vi "PicoScope4000aSettings.vi"(0 "handle in":i16=16384, 3 "Trigger Settings":T3={"Trigger Enabled"=FALSE, "Trigger Source"=enum."Channel A", "Trigger Threshold (Volts/Probe units)"=0.0, "Trigger Direction"=2, "Trigger Delay (samples)"=0, "Auto Trigger Time (ms)"=1000} {"Trigger Direction" items=["Above", "Below", "Rising", "Falling", "Rising or Falling"]}, 4 "Max ADC value":i16=32767, 5 "error in":errorcluster, 6 "Channel A Settings":T2={"Enabled"=FALSE, "Coupling"=1, "Range"=6, "Analogue Offset"=0.0, "Bandwidth Limit"=0} {"Bandwidth Limit" items=["Full", "20kHz", "100kHz", "1MHz"]; "Range" items=["10 mV", "20 mV", "50 mV", "100 mV", "200 mV", "500 mV", "1 V", "2 V", "5 V", "10 V", "20 V", "50 V ", "100 V"]; "Coupling" items=["AC", "DC"]}, 7 "Channel E Settings":T2={"Enabled"=FALSE, "Coupling"=1, "Range"=6, "Analogue Offset"=0.0, "Bandwidth Limit"=0} {"Bandwidth Limit" items=["Full", "20kHz", "100kHz", "1MHz"]; "Range" items=["10 mV", "20 mV", "50 mV", "100 mV", "200 mV", "500 mV", "1 V", "2 V", "5 V", "10 V", "20 V", "50 V ", "100 V"]; "Coupling" items=["AC", "DC"]}, 8 "Channel B Settings":T2={"Enabled"=FALSE, "Coupling"=1, "Range"=6, "Analogue Offset"=0.0, "Bandwidth Limit"=0} {"Bandwidth Limit" items=["Full", "20kHz", "100kHz", "1MHz"]; "Range" items=["10 mV", "20 mV", "50 mV", "100 mV", "200 mV", "500 mV", "1 V", "2 V", "5 V", "10 V", "20 V", "50 V ", "100 V"]; "Coupling" items=["AC", "DC"]}, 9 "Channel F Settings":T2={"Enabled"=FALSE, "Coupling"=1, "Range"=6, "Analogue Offset"=0.0, "Bandwidth Limit"=0} {"Bandwidth Limit" items=["Full", "20kHz", "100kHz", "1MHz"]; "Range" items=["10 mV", "20 mV", "50 mV", "100 mV", "200 mV", "500 mV", "1 V", "2 V", "5 V", "10 V", "20 V", "50 V ", "100 V"]; "Coupling" items=["AC", "DC"]}, 10 "Channel C Settings":T2={"Enabled"=FALSE, "Coupling"=1, "Range"=6, "Analogue Offset"=0.0, "Bandwidth Limit"=0} {"Bandwidth Limit" items=["Full", "20kHz", "100kHz", "1MHz"]; "Range" items=["10 mV", "20 mV", "50 mV", "100 mV", "200 mV", "500 mV", "1 V", "2 V", "5 V", "10 V", "20 V", "50 V ", "100 V"]; "Coupling" items=["AC", "DC"]}, 11 "Channel G Settings":T2={"Enabled"=FALSE, "Coupling"=1, "Range"=6, "Analogue Offset"=0.0, "Bandwidth Limit"=0} {"Bandwidth Limit" items=["Full", "20kHz", "100kHz", "1MHz"]; "Range" items=["10 mV", "20 mV", "50 mV", "100 mV", "200 mV", "500 mV", "1 V", "2 V", "5 V", "10 V", "20 V", "50 V ", "100 V"]; "Coupling" items=["AC", "DC"]}, 12 "Channel D Settings":T2={"Enabled"=FALSE, "Coupling"=1, "Range"=6, "Analogue Offset"=0.0, "Bandwidth Limit"=0} {"Bandwidth Limit" items=["Full", "20kHz", "100kHz", "1MHz"]; "Range" items=["10 mV", "20 mV", "50 mV", "100 mV", "200 mV", "500 mV", "1 V", "2 V", "5 V", "10 V", "20 V", "50 V ", "100 V"]; "Coupling" items=["AC", "DC"]}, 13 "Channel H Settings":T2={"Enabled"=FALSE, "Coupling"=1, "Range"=6, "Analogue Offset"=0.0, "Bandwidth Limit"=0} {"Bandwidth Limit" items=["Full", "20kHz", "100kHz", "1MHz"]; "Range" items=["10 mV", "20 mV", "50 mV", "100 mV", "200 mV", "500 mV", "1 V", "2 V", "5 V", "10 V", "20 V", "50 V ", "100 V"]; "Coupling" items=["AC", "DC"]}, 18 "Unit Info":T1={"Driver Version"="2.1.82.3072", "USB Version"="2.0", "Hardware"="1", "Variant"="4444", "Batch and Serial"="ET311/0003", "Cal Date"="24Jan17", "Kernel Version"="1.0", "Digital HW Version"="1", "Analogue HW Version"="1", "Firmware 1"="1.7.5.0", "Firmware 2"="1.1.6.0", "Num. channels"=4}) -> (14 "handle out":i16=16384, 16 "Enabled array":i16[](array[numeric])=[1, 0, 0, 0, 0, 0, 0, 0], 19 "error out":errorcluster)   [LabVIEW 2010]
doc: "This VI is used to set up the oscilloscope. The inputs are clusters for setting channel and simple trigger settings. Advanced triggers can be set up using PicoScope3000aAdvancedTriggerSettings.vi"
uses:
  Program Files/Pico Technology/SDK/lib/ps4000a.dll
  PicoScope4000aAnalogChannelSettings.ctl
panel:
  # "Note Bandwith Limit not avaiable on all models"
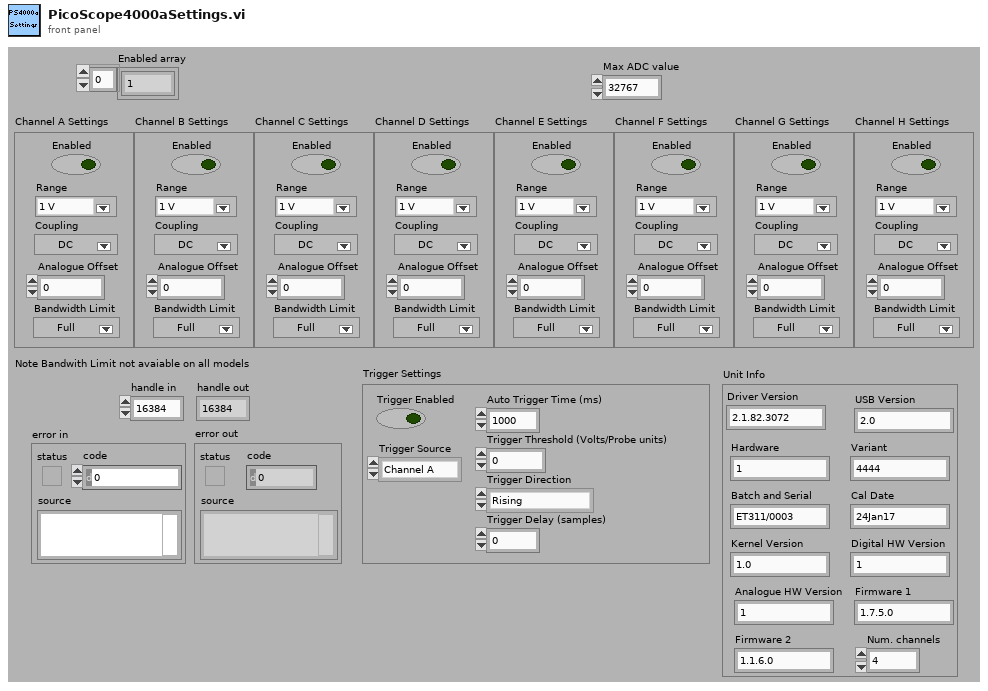
[diagram p1: front panel]
types:
  T1 = cluster{"Driver Version":string, "USB Version":string, "Hardware":string, "Variant":string, "Batch and Serial":string, "Cal Date":string, "Kernel Version":string, "Digital HW Version":string, "Analogue HW Version":string, "Firmware 1":string, "Firmware 2":string, "Num. channels":i16}
  T2 = typedef "PicoScope4000aAnalogChannelSettings.ctl" = cluster{"Enabled":bool, "Coupling":i16, "Range":u32, "Analogue Offset":sgl, "Bandwidth Limit":u32}
  T3 = cluster{"Trigger Enabled":bool, "Trigger Source":enum16{"Channel A", "Channel B", "Channel C", "Channel D", "Channel E", "Channel F", "Channel G", "Channel H"}, "Trigger Threshold (Volts/Probe units)":dbl, "Trigger Direction":u16, "Trigger Delay (samples)":u32, "Auto Trigger Time (ms)":i16}
  T4 = enum16{"Channel A", "Channel B", "Channel C", "Channel D", "Channel E", "Channel F", "Channel G", "Channel H"}
  T5 = cluster{"status":bool, "code":u32, "source":string}
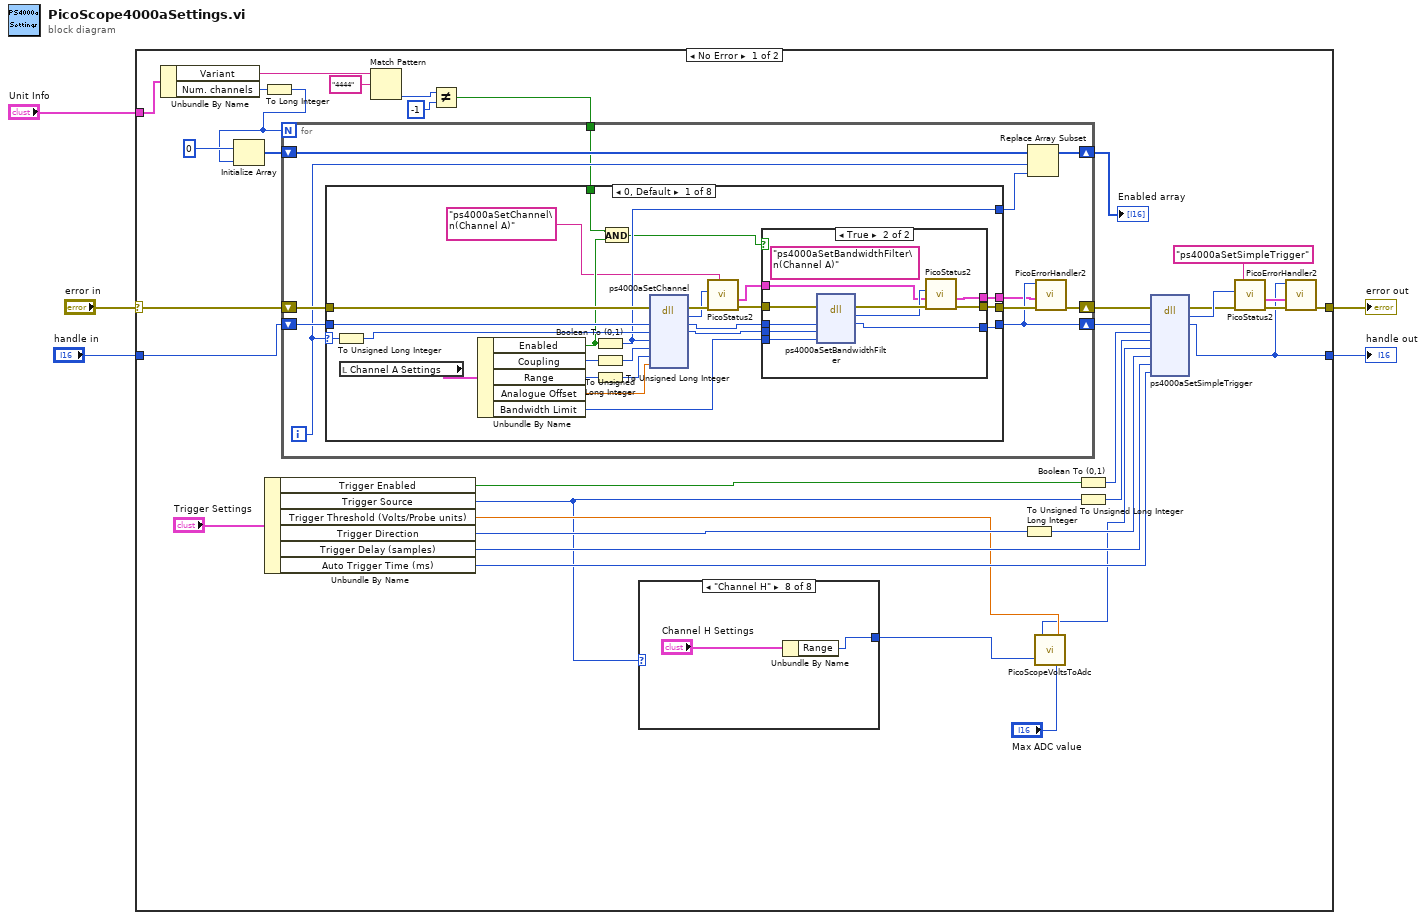
[diagram p0: block diagram]
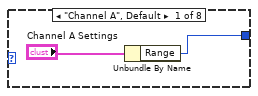
[diagram p2: hidden frame]
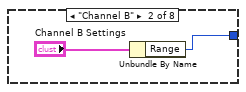
[diagram p3: hidden frame]
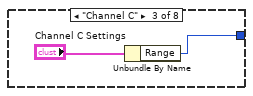
[diagram p4: hidden frame]
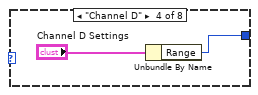
[diagram p5: hidden frame]
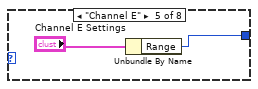
[diagram p6: hidden frame]
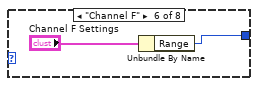
[diagram p7: hidden frame]
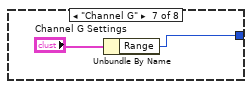
[diagram p8: hidden frame]
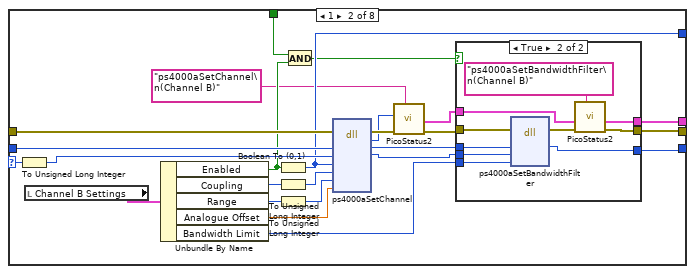
[diagram p10: hidden frame]
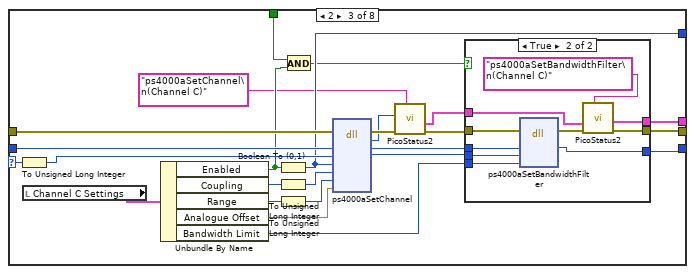
[diagram p12: hidden frame]
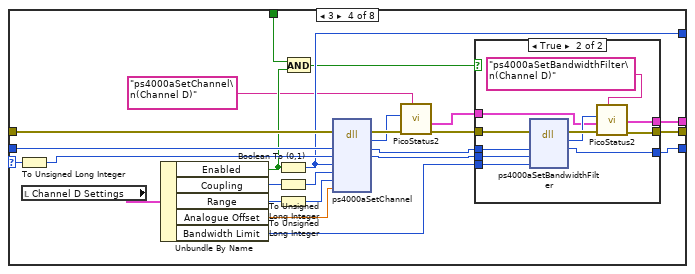
[diagram p14: hidden frame]
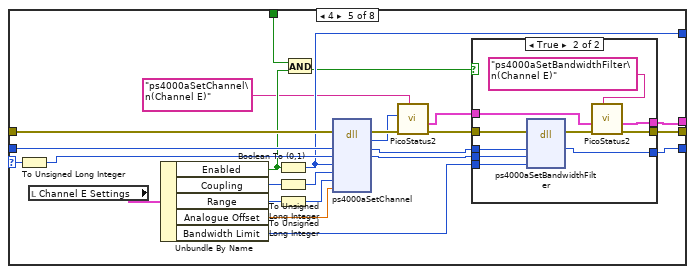
[diagram p16: hidden frame]
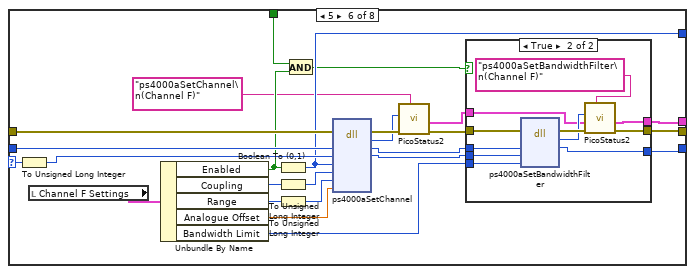
[diagram p18: hidden frame]
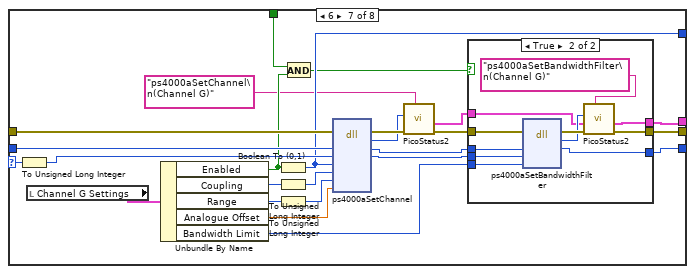
[diagram p20: hidden frame]
diagram:
  n1 = case shown="No Error" "error in" {
    selector: "error in" -> [w26 w377]
    tunnel: "handle in" -> [w29 w376]
    tunnel: [w6 w376] -> w3
    tunnel: [w8 w377] -> w2
    tunnel: "Unit Info" -> [w22 _]
    frame No Error {
      n2 = Unbundle By Name(w22) -> ("Variant"=w16:string, "Num. channels"=w11:i16)
      n3 = To Long Integer(number=w11) -> (32bit integer=w10:i32)
      n4 = Initialize Array(i16 0 ("element"), w10) -> (w24:i16[])
      n5 = Unbundle By Name("Trigger Settings") -> ("Trigger Enabled"=w34:bool, "Trigger Source"=w18:T4, "Trigger Threshold (Volts/Probe units)"=w20:dbl, "Trigger Direction"=w37:u16, "Trigger Delay (samples)"=w36:u32, "Auto Trigger Time (ms)"=w35:i16)
      n6 = Match Pattern(string=w16, regular expression="4444") -> (offset past match=w14:i32)  [unwired: 1 in, 3 out]
      n7 = Not Equal?(x=w14, y=-1) -> (x != y?=w12:bool)
      n8 = for {
        N: w10 -> [_]
        shift-right: [w60] -> w28
        shift-left: w26 -> [w66]
        shift-right: [w59] -> w27
        shift-left: w29 -> [w67]
        shift-right: [w62] -> w23
        shift-left: w24 -> [w63]
        tunnel: w12 -> [w58]
        i -> [w65]
        n9 = case shown="0, Default" w65 {
          selector: w65 -> [w89 w123 w159 w198 w237 w275 w313 w353]
          tunnel: w67 -> [w90 w121 w161 w199 w238 w276 w315 w354]
          tunnel: [w80 w116 w157 w195 w234 w269 w311 w350] -> w61
          tunnel: w66 -> [w92 w122 w162 w200 w239 w277 w316 w355]
          tunnel: [w79 w115 w156 w194 w233 w268 w310 w349] -> w59
          tunnel: [w82 w120 w158 w196 w235 w273 w312 w351] -> w64
          tunnel: w58 -> [w75 w112 w150 w188 w227 w265 w305 w343]
          tunnel: [w68 w108 w146 w184 w224 w260 w299 w338] -> w57
          frame 0, Default {
            n10 = To Unsigned Long Integer(number=w89) -> (unsigned 32bit integer=w83:u32)
            n11 = local read "Channel A Settings"() -> (w91:T2)
            n12 = Unbundle By Name(w91) -> ("Enabled"=w74:bool, "Coupling"=w88:i16, "Range"=w87:u32, "Analogue Offset"=w86:sgl, "Bandwidth Limit"=w77:u32)
            n13 = Boolean To (0,1)(Boolean=w74) -> (0, 1=w82:i16)
            n14 = To Unsigned Long Integer(number=w88) -> (unsigned 32bit integer=w84:u32)
            n15 = To Unsigned Long Integer(number=w87) -> (unsigned 32bit integer=w85:u32)
            n16 = And(x=w75, y=w74) -> (x .and. y?=w76:bool)
            n17 = dll-call lib="/Program Files/Pico Technology/SDK/lib/ps4000a.dll" fn="ps4000aSetChannel" ("ps3000.dll:_ps3000_open_unit@0")(error in=w92, "handle"=w90, "channel"=w83, "enabled"=w82, "dc"=w84, "range"=w85, "analogueOffset"=w86) -> (error out=w73:errorcluster, "PICO_STATUS"=w71:u32, "handle"=w81:i16, "channel"=w78:u32)  [unwired: 6 in, 1 out]
            n18 = call "PicoStatus2.vi"("PICO source"="ps4000aSetChannel\n(Channel A)" ("source"), "Error in"=w73, "PICO STATUS"=w71) -> ("error out"=w70:errorcluster, "PICO_STATUS out"=w69:T5)  [unwired: 5 in]
            n19 = case shown="True" w76 {
              tunnel: w70 -> [w95 w105]
              tunnel: w81 -> [w94 w104]
              tunnel: [w95 w99] -> w80
              tunnel: [w94 w103] -> w79
              tunnel: w78 -> [_ w102]
              tunnel: w77 -> [_ w101]
              tunnel: w69 -> [w93 w97]
              tunnel: [w93 w96] -> w68
              frame False {
              }
              frame True {
                (unwired) "ps4000aSetBandwidthFilter\n(Channel A)" ("source")
                n20 = dll-call lib="/Program Files/Pico Technology/SDK/lib/ps4000a.dll" fn="ps4000aSetBandwidthFilter" ("ps3000.dll:_ps3000_open_unit@0")(error in=w105, "handle"=w104, "channel"=w102, "bandwidth"=w101) -> (error out=w100:errorcluster, "PICO_STATUS"=w98:u32, "handle"=w103:i16)  [unwired: 4 in, 1 out]
                n21 = call "PicoStatus2.vi"("Error in"=w100, "PICO_STATUS in"=w97, "PICO STATUS"=w98) -> ("error out"=w99:errorcluster, "PICO_STATUS out"=w96:T5)  [unwired: 5 in]
              }
            }
          }
          frame 1 {
            n22 = To Unsigned Long Integer(number=w123) -> (unsigned 32bit integer=w125:u32)
            n23 = local read "Channel B Settings"() -> (w124:T2)
            n24 = Unbundle By Name(w124) -> ("Enabled"=w113:bool, "Coupling"=w130:i16, "Range"=w129:u32, "Analogue Offset"=w128:sgl, "Bandwidth Limit"=w117:u32)
            n25 = Boolean To (0,1)(Boolean=w113) -> (0, 1=w120:i16)
            n26 = To Unsigned Long Integer(number=w130) -> (unsigned 32bit integer=w126:u32)
            n27 = To Unsigned Long Integer(number=w129) -> (unsigned 32bit integer=w127:u32)
            n28 = And(x=w112, y=w113) -> (x .and. y?=w114:bool)
            n29 = dll-call lib="/Program Files/Pico Technology/SDK/lib/ps4000a.dll" fn="ps4000aSetChannel" ("ps3000.dll:_ps3000_open_unit@0")(error in=w122, "handle"=w121, "channel"=w125, "enabled"=w120, "dc"=w126, "range"=w127, "analogueOffset"=w128) -> (error out=w111:errorcluster, "PICO_STATUS"=w110:u32, "handle"=w119:i16, "channel"=w118:u32)  [unwired: 6 in, 1 out]
            n30 = call "PicoStatus2.vi"("PICO source"="ps4000aSetChannel\n(Channel B)" ("source"), "Error in"=w111, "PICO STATUS"=w110) -> ("error out"=w109:errorcluster, "PICO_STATUS out"=w107:T5)  [unwired: 5 in]
            n31 = case shown="True" w114 {
              tunnel: w109 -> [w133 w143]
              tunnel: w119 -> [w132 w142]
              tunnel: [w133 w137] -> w116
              tunnel: [w132 w141] -> w115
              tunnel: w118 -> [_ w140]
              tunnel: w117 -> [_ w139]
              tunnel: [w131 w136] -> w108
              tunnel: w107 -> [w131 w135]
              frame False {
              }
              frame True {
                n32 = dll-call lib="/Program Files/Pico Technology/SDK/lib/ps4000a.dll" fn="ps4000aSetBandwidthFilter" ("ps3000.dll:_ps3000_open_unit@0")(error in=w143, "handle"=w142, "channel"=w140, "bandwidth"=w139) -> (error out=w138:errorcluster, "handle"=w141:i16)  [unwired: 5 in, 1 out]
                n33 = call "PicoStatus2.vi"("PICO source"="ps4000aSetBandwidthFilter\n(Channel B)" ("source"), "Error in"=w138, "PICO_STATUS in"=w135) -> ("error out"=w137:errorcluster, "PICO_STATUS out"=w136:T5)  [unwired: 5 in]
              }
            }
          }
          frame 2 {
            n34 = To Unsigned Long Integer(number=w159) -> (unsigned 32bit integer=w163:u32)
            n35 = local read "Channel C Settings"() -> (w160:T2)
            n36 = Unbundle By Name(w160) -> ("Enabled"=w151:bool, "Coupling"=w168:i16, "Range"=w167:u32, "Analogue Offset"=w166:sgl, "Bandwidth Limit"=w153:u32)
            n37 = Boolean To (0,1)(Boolean=w151) -> (0, 1=w158:i16)
            n38 = To Unsigned Long Integer(number=w168) -> (unsigned 32bit integer=w164:u32)
            n39 = To Unsigned Long Integer(number=w167) -> (unsigned 32bit integer=w165:u32)
            n40 = And(x=w150, y=w151) -> (x .and. y?=w152:bool)
            n41 = dll-call lib="/Program Files/Pico Technology/SDK/lib/ps4000a.dll" fn="ps4000aSetChannel" ("ps3000.dll:_ps3000_open_unit@0")(error in=w162, "handle"=w161, "channel"=w163, "enabled"=w158, "dc"=w164, "range"=w165, "analogueOffset"=w166) -> (error out=w149:errorcluster, "PICO_STATUS"=w148:u32, "handle"=w155:i16, "channel"=w154:u32)  [unwired: 6 in, 1 out]
            n42 = call "PicoStatus2.vi"("PICO source"="ps4000aSetChannel\n(Channel C)" ("source"), "Error in"=w149, "PICO STATUS"=w148) -> ("error out"=w147:errorcluster, "PICO_STATUS out"=w144:T5)  [unwired: 5 in]
            n43 = case shown="True" w152 {
              tunnel: w147 -> [w171 w181]
              tunnel: w155 -> [w170 w180]
              tunnel: [w171 w175] -> w157
              tunnel: [w170 w179] -> w156
              tunnel: w154 -> [_ w178]
              tunnel: w153 -> [_ w177]
              tunnel: [w169 w174] -> w146
              tunnel: w144 -> [w169 w172]
              frame False {
              }
              frame True {
                n44 = dll-call lib="/Program Files/Pico Technology/SDK/lib/ps4000a.dll" fn="ps4000aSetBandwidthFilter" ("ps3000.dll:_ps3000_open_unit@0")(error in=w181, "handle"=w180, "channel"=w178, "bandwidth"=w177) -> (error out=w176:errorcluster, "handle"=w179:i16)  [unwired: 5 in, 1 out]
                n45 = call "PicoStatus2.vi"("PICO source"="ps4000aSetBandwidthFilter\n(Channel C)" ("source"), "Error in"=w176, "PICO_STATUS in"=w172) -> ("error out"=w175:errorcluster, "PICO_STATUS out"=w174:T5)  [unwired: 5 in]
              }
            }
          }
          frame 3 {
            n46 = To Unsigned Long Integer(number=w198) -> (unsigned 32bit integer=w201:u32)
            n47 = local read "Channel D Settings"() -> (w197:T2)
            n48 = Unbundle By Name(w197) -> ("Enabled"=w189:bool, "Coupling"=w206:i16, "Range"=w205:u32, "Analogue Offset"=w204:sgl, "Bandwidth Limit"=w191:u32)
            n49 = Boolean To (0,1)(Boolean=w189) -> (0, 1=w196:i16)
            n50 = To Unsigned Long Integer(number=w206) -> (unsigned 32bit integer=w202:u32)
            n51 = To Unsigned Long Integer(number=w205) -> (unsigned 32bit integer=w203:u32)
            n52 = And(x=w188, y=w189) -> (x .and. y?=w190:bool)
            n53 = dll-call lib="/Program Files/Pico Technology/SDK/lib/ps4000a.dll" fn="ps4000aSetChannel" ("ps3000.dll:_ps3000_open_unit@0")(error in=w200, "handle"=w199, "channel"=w201, "enabled"=w196, "dc"=w202, "range"=w203, "analogueOffset"=w204) -> (error out=w187:errorcluster, "PICO_STATUS"=w186:u32, "handle"=w193:i16, "channel"=w192:u32)  [unwired: 6 in, 1 out]
            n54 = call "PicoStatus2.vi"("PICO source"="ps4000aSetChannel\n(Channel D)" ("source"), "Error in"=w187, "PICO STATUS"=w186) -> ("error out"=w185:errorcluster, "PICO_STATUS out"=w182:T5)  [unwired: 5 in]
            n55 = case shown="True" w190 {
              tunnel: w185 -> [w209 w220]
              tunnel: w193 -> [w208 w219]
              tunnel: [w209 w214] -> w195
              tunnel: [w208 w218] -> w194
              tunnel: w192 -> [_ w217]
              tunnel: w191 -> [_ w216]
              tunnel: [w207 w213] -> w184
              tunnel: w182 -> [w207 w210]
              frame False {
              }
              frame True {
                n56 = dll-call lib="/Program Files/Pico Technology/SDK/lib/ps4000a.dll" fn="ps4000aSetBandwidthFilter" ("ps3000.dll:_ps3000_open_unit@0")(error in=w220, "handle"=w219, "channel"=w217, "bandwidth"=w216) -> (error out=w215:errorcluster, "PICO_STATUS"=w212:u32, "handle"=w218:i16)  [unwired: 4 in, 1 out]
                n57 = call "PicoStatus2.vi"("PICO source"="ps4000aSetBandwidthFilter\n(Channel D)" ("source"), "Error in"=w215, "PICO_STATUS in"=w210, "PICO STATUS"=w212) -> ("error out"=w214:errorcluster, "PICO_STATUS out"=w213:T5)  [unwired: 4 in]
              }
            }
          }
          frame 4 {
            n58 = To Unsigned Long Integer(number=w237) -> (unsigned 32bit integer=w240:u32)
            n59 = local read "Channel E Settings"() -> (w236:T2)
            n60 = Unbundle By Name(w236) -> ("Enabled"=w228:bool, "Coupling"=w245:i16, "Range"=w244:u32, "Analogue Offset"=w243:sgl, "Bandwidth Limit"=w230:u32)
            n61 = Boolean To (0,1)(Boolean=w228) -> (0, 1=w235:i16)
            n62 = To Unsigned Long Integer(number=w245) -> (unsigned 32bit integer=w241:u32)
            n63 = To Unsigned Long Integer(number=w244) -> (unsigned 32bit integer=w242:u32)
            n64 = And(x=w227, y=w228) -> (x .and. y?=w229:bool)
            n65 = dll-call lib="/Program Files/Pico Technology/SDK/lib/ps4000a.dll" fn="ps4000aSetChannel" ("ps3000.dll:_ps3000_open_unit@0")(error in=w239, "handle"=w238, "channel"=w240, "enabled"=w235, "dc"=w241, "range"=w242, "analogueOffset"=w243) -> (error out=w226:errorcluster, "PICO_STATUS"=w223:u32, "handle"=w232:i16, "channel"=w231:u32)  [unwired: 6 in, 1 out]
            n66 = call "PicoStatus2.vi"("PICO source"="ps4000aSetChannel\n(Channel E)" ("source"), "Error in"=w226, "PICO STATUS"=w223) -> ("error out"=w225:errorcluster, "PICO_STATUS out"=w221:T5)  [unwired: 5 in]
            n67 = case shown="True" w229 {
              tunnel: w225 -> [w248 w258]
              tunnel: w232 -> [w247 w257]
              tunnel: [w248 w252] -> w234
              tunnel: [w247 w256] -> w233
              tunnel: w231 -> [_ w255]
              tunnel: w230 -> [_ w254]
              tunnel: [w246 w250] -> w224
              tunnel: w221 -> [w246 w249]
              frame False {
              }
              frame True {
                n68 = dll-call lib="/Program Files/Pico Technology/SDK/lib/ps4000a.dll" fn="ps4000aSetBandwidthFilter" ("ps3000.dll:_ps3000_open_unit@0")(error in=w258, "handle"=w257, "channel"=w255, "bandwidth"=w254) -> (error out=w253:errorcluster, "handle"=w256:i16)  [unwired: 5 in, 1 out]
                n69 = call "PicoStatus2.vi"("PICO source"="ps4000aSetBandwidthFilter\n(Channel E)" ("source"), "Error in"=w253, "PICO_STATUS in"=w249) -> ("error out"=w252:errorcluster, "PICO_STATUS out"=w250:T5)  [unwired: 5 in]
              }
            }
          }
          frame 5 {
            n70 = To Unsigned Long Integer(number=w275) -> (unsigned 32bit integer=w278:u32)
            n71 = local read "Channel F Settings"() -> (w274:T2)
            n72 = Unbundle By Name(w274) -> ("Enabled"=w266:bool, "Coupling"=w283:i16, "Range"=w282:u32, "Analogue Offset"=w281:sgl, "Bandwidth Limit"=w270:u32)
            n73 = Boolean To (0,1)(Boolean=w266) -> (0, 1=w273:i16)
            n74 = To Unsigned Long Integer(number=w283) -> (unsigned 32bit integer=w279:u32)
            n75 = To Unsigned Long Integer(number=w282) -> (unsigned 32bit integer=w280:u32)
            n76 = And(x=w265, y=w266) -> (x .and. y?=w267:bool)
            n77 = dll-call lib="/Program Files/Pico Technology/SDK/lib/ps4000a.dll" fn="ps4000aSetChannel" ("ps3000.dll:_ps3000_open_unit@0")(error in=w277, "handle"=w276, "channel"=w278, "enabled"=w273, "dc"=w279, "range"=w280, "analogueOffset"=w281) -> (error out=w264:errorcluster, "PICO_STATUS"=w262:u32, "handle"=w272:i16, "channel"=w271:u32)  [unwired: 6 in, 1 out]
            n78 = call "PicoStatus2.vi"("PICO source"="ps4000aSetChannel\n(Channel F)" ("source"), "Error in"=w264, "PICO STATUS"=w262) -> ("error out"=w261:errorcluster, "PICO_STATUS out"=w259:T5)  [unwired: 5 in]
            n79 = case shown="True" w267 {
              tunnel: w261 -> [w286 w297]
              tunnel: w272 -> [w285 w296]
              tunnel: [w286 w290] -> w269
              tunnel: [w285 w295] -> w268
              tunnel: w271 -> [_ w294]
              tunnel: w270 -> [_ w293]
              tunnel: [w284 w289] -> w260
              tunnel: w259 -> [w284 w287]
              frame False {
              }
              frame True {
                n80 = dll-call lib="/Program Files/Pico Technology/SDK/lib/ps4000a.dll" fn="ps4000aSetBandwidthFilter" ("ps3000.dll:_ps3000_open_unit@0")(error in=w297, "handle"=w296, "channel"=w294, "bandwidth"=w293) -> (error out=w292:errorcluster, "PICO_STATUS"=w291:u32, "handle"=w295:i16)  [unwired: 4 in, 1 out]
                n81 = call "PicoStatus2.vi"("PICO source"="ps4000aSetBandwidthFilter\n(Channel F)" ("source"), "Error in"=w292, "PICO_STATUS in"=w287, "PICO STATUS"=w291) -> ("error out"=w290:errorcluster, "PICO_STATUS out"=w289:T5)  [unwired: 4 in]
              }
            }
          }
          frame 6 {
            n82 = To Unsigned Long Integer(number=w313) -> (unsigned 32bit integer=w317:u32)
            n83 = local read "Channel G Settings"() -> (w314:T2)
            n84 = Unbundle By Name(w314) -> ("Enabled"=w306:bool, "Coupling"=w322:i16, "Range"=w321:u32, "Analogue Offset"=w320:sgl, "Bandwidth Limit"=w307:u32)
            n85 = Boolean To (0,1)(Boolean=w306) -> (0, 1=w312:i16)
            n86 = To Unsigned Long Integer(number=w322) -> (unsigned 32bit integer=w318:u32)
            n87 = To Unsigned Long Integer(number=w321) -> (unsigned 32bit integer=w319:u32)
            n88 = And(x=w305, y=w306) -> (x .and. y?=w304:bool)
            n89 = dll-call lib="/Program Files/Pico Technology/SDK/lib/ps4000a.dll" fn="ps4000aSetChannel" ("ps3000.dll:_ps3000_open_unit@0")(error in=w316, "handle"=w315, "channel"=w317, "enabled"=w312, "dc"=w318, "range"=w319, "analogueOffset"=w320) -> (error out=w303:errorcluster, "PICO_STATUS"=w301:u32, "handle"=w309:i16, "channel"=w308:u32)  [unwired: 6 in, 1 out]
            n90 = call "PicoStatus2.vi"("PICO source"="ps4000aSetChannel\n(Channel G)" ("source"), "Error in"=w303, "PICO STATUS"=w301) -> ("error out"=w300:errorcluster, "PICO_STATUS out"=w298:T5)  [unwired: 5 in]
            n91 = case shown="True" w304 {
              tunnel: w300 -> [w325 w336]
              tunnel: w309 -> [w324 w335]
              tunnel: [w325 w329] -> w311
              tunnel: [w324 w334] -> w310
              tunnel: w308 -> [_ w333]
              tunnel: w307 -> [_ w332]
              tunnel: [w323 w327] -> w299
              tunnel: w298 -> [w323 w326]
              frame False {
              }
              frame True {
                n92 = dll-call lib="/Program Files/Pico Technology/SDK/lib/ps4000a.dll" fn="ps4000aSetBandwidthFilter" ("ps3000.dll:_ps3000_open_unit@0")(error in=w336, "handle"=w335, "channel"=w333, "bandwidth"=w332) -> (error out=w331:errorcluster, "PICO_STATUS"=w330:u32, "handle"=w334:i16)  [unwired: 4 in, 1 out]
                n93 = call "PicoStatus2.vi"("PICO source"="ps4000aSetBandwidthFilter\n(Channel G)" ("source"), "Error in"=w331, "PICO_STATUS in"=w326, "PICO STATUS"=w330) -> ("error out"=w329:errorcluster, "PICO_STATUS out"=w327:T5)  [unwired: 4 in]
              }
            }
          }
          frame 7 {
            n94 = To Unsigned Long Integer(number=w353) -> (unsigned 32bit integer=w356:u32)
            n95 = local read "Channel H Settings"() -> (w352:T2)
            n96 = Unbundle By Name(w352) -> ("Enabled"=w344:bool, "Coupling"=w361:i16, "Range"=w360:u32, "Analogue Offset"=w359:sgl, "Bandwidth Limit"=w346:u32)
            n97 = Boolean To (0,1)(Boolean=w344) -> (0, 1=w351:i16)
            n98 = To Unsigned Long Integer(number=w361) -> (unsigned 32bit integer=w357:u32)
            n99 = To Unsigned Long Integer(number=w360) -> (unsigned 32bit integer=w358:u32)
            n100 = And(x=w343, y=w344) -> (x .and. y?=w345:bool)
            n101 = dll-call lib="/Program Files/Pico Technology/SDK/lib/ps4000a.dll" fn="ps4000aSetChannel" ("ps3000.dll:_ps3000_open_unit@0")(error in=w355, "handle"=w354, "channel"=w356, "enabled"=w351, "dc"=w357, "range"=w358, "analogueOffset"=w359) -> (error out=w342:errorcluster, "PICO_STATUS"=w341:u32, "handle"=w348:i16, "channel"=w347:u32)  [unwired: 6 in, 1 out]
            n102 = call "PicoStatus2.vi"("PICO source"="ps4000aSetChannel\n(Channel H)" ("source"), "Error in"=w342, "PICO STATUS"=w341) -> ("error out"=w339:errorcluster, "PICO_STATUS out"=w337:T5)  [unwired: 5 in]
            n103 = case shown="True" w345 {
              tunnel: w339 -> [w364 w375]
              tunnel: w348 -> [w363 w374]
              tunnel: [w364 w369] -> w350
              tunnel: [w363 w373] -> w349
              tunnel: w347 -> [_ w372]
              tunnel: w346 -> [_ w371]
              tunnel: [w362 w368] -> w338
              tunnel: w337 -> [w362 w365]
              frame False {
              }
              frame True {
                n104 = dll-call lib="/Program Files/Pico Technology/SDK/lib/ps4000a.dll" fn="ps4000aSetBandwidthFilter" ("ps3000.dll:_ps3000_open_unit@0")(error in=w375, "handle"=w374, "channel"=w372, "bandwidth"=w371) -> (error out=w370:errorcluster, "PICO_STATUS"=w367:u32, "handle"=w373:i16)  [unwired: 4 in, 1 out]
                n105 = call "PicoStatus2.vi"("PICO source"="ps4000aSetBandwidthFilter\n(Channel H)" ("source"), "Error in"=w370, "PICO_STATUS in"=w365, "PICO STATUS"=w367) -> ("error out"=w369:errorcluster, "PICO_STATUS out"=w368:T5)  [unwired: 4 in]
              }
            }
          }
        }
        n106 = Replace Array Subset(array=w63, new element=w64, index=w65) -> (w62:i16[])
        n107 = call "PicoErrorHandler2.vi"("error in (no error)"=w61, "PICO_STATUS in"=w57, "handle In"=w59) -> ("error out"=w60:errorcluster)  [unwired: 8 in]
      }
      "Enabled array" <- w23
      n108 = case shown="\"Channel H\"" w18 {
        tunnel: [w41 w43 w45 w47 w49 w51 w53 w55] -> w17
        frame "Channel A", Default {
          n109 = Unbundle By Name("Channel A Settings") -> ("Range"=w41:u32)
        }
        frame "Channel B" {
          n110 = Unbundle By Name("Channel B Settings") -> ("Range"=w43:u32)
        }
        frame "Channel C" {
          n111 = Unbundle By Name("Channel C Settings") -> ("Range"=w45:u32)
        }
        frame "Channel D" {
          n112 = Unbundle By Name("Channel D Settings") -> ("Range"=w47:u32)
        }
        frame "Channel E" {
          n113 = Unbundle By Name("Channel E Settings") -> ("Range"=w49:u32)
        }
        frame "Channel F" {
          n114 = Unbundle By Name("Channel F Settings") -> ("Range"=w51:u32)
        }
        frame "Channel G" {
          n115 = Unbundle By Name("Channel G Settings") -> ("Range"=w53:u32)
        }
        frame "Channel H" {
          n116 = Unbundle By Name("Channel H Settings") -> ("Range"=w55:u32)
        }
      }
      n117 = To Unsigned Long Integer(number=w37) -> (unsigned 32bit integer=w39:u32)
      n118 = call "PicoScopeVoltsToAdc.vi"("Max_adc"="Max ADC value", "Units"=w20, "Range Index"=w17) -> ("ADC count"=w19:i16)
      n119 = Boolean To (0,1)(Boolean=w34) -> (0, 1=w33:i16)
      n120 = To Unsigned Long Integer(number=w18) -> (unsigned 32bit integer=w40:u32)
      n121 = dll-call lib="/Program Files/Pico Technology/SDK/lib/ps4000a.dll" fn="ps4000aSetSimpleTrigger" ("ps3000.dll:_ps3000_open_unit@0")(error in=w28, "handle"=w27, "enable"=w33, "source"=w40, "threshold"=w19, "direction"=w39, "delay"=w36, "autoTrigger_ms"=w35) -> (error out=w31:errorcluster, "PICO_STATUS"=w32:u32, "handle"=w6:i16)  [unwired: 8 in, 1 out]
      n122 = call "PicoStatus2.vi"("PICO source"="ps4000aSetSimpleTrigger" ("source"), "Error in"=w31, "PICO STATUS"=w32) -> ("error out"=w9:errorcluster, "PICO_STATUS out"=w7:T5)  [unwired: 5 in]
      n123 = call "PicoErrorHandler2.vi"("error in (no error)"=w9, "PICO_STATUS in"=w7, "handle In"=w6) -> ("error out"=w8:errorcluster)  [unwired: 8 in]
    }
    frame Error {
    }
  }
  "handle out" <- w3
  "error out" <- w2
